vi "Incorporate New Data.vi"(8 "error in (no error)":errorcluster, 10 "New Graph Data":waveform(dbl)[](array[waveform]), 11 "Data in":T1={"UI References"={"Exit Ref"=refnum, "Save Ref"=refnum, "Open Ref"=refnum, "Export Ref"=refnum, "Acquire Ref"=refnum, "Configure Ref"=refnum, "Graph Ref"=refnum, "Clear Ref"=refnum, "Analyze Ref"=refnum, "Status Ref"=refnum, "Snapshot Ref"=refnum}, "User Specified"={"Hardware Configuration"={"VGC50"={"serial settings"={"port"="", "baud rate"=115200}, "device information"={"type"="", "model number"="", "serial number"="", "firmware version"="", "hardware version"=""}, "gauges"=[], "VGC"=refnum, "Backing SP"={"mode"=0, "thresholds"={"lower"=0.0, "upper"=0.0}, "on"=FALSE}, "Chamber SP"={"mode"=0, "thresholds"={"lower"=0.0, "upper"=0.0}, "on"=FALSE}}, "PTC10"={"serial settings"={"port"="", "baud rate"=0}, "PTC10 Info"={"Manufacturer"="", "Instrument"="", "Serial Number"="", "Firmware"=""}, "VISA resource name"=""}}, "New Data Behavior"=enum."Replace", "Vacuum Graph config"={"Log/Lin"=TRUE, "Show Backing"=FALSE, "Show Chamber"=FALSE}}} {"User Specified"."Hardware Configuration"."PTC10"."serial settings"."baud rate" items=["9600"=9600, "19200"=19200, "38400"=38400, "57600"=57600, "115200"=115200]; "User Specified"."Hardware Configuration"."VGC50"."Chamber SP"."thresholds"."upper" format="%#_5p"; "User Specified"."Hardware Configuration"."VGC50"."Chamber SP"."thresholds"."lower" format="%#_5p"; "User Specified"."Hardware Configuration"."VGC50"."Chamber SP"."mode" items=["off", "on", "channel 1", "channel 2", "channel 3"]; "User Specified"."Hardware Configuration"."VGC50"."Backing SP"."thresholds"."upper" format="%#_5p"; "User Specified"."Hardware Configuration"."VGC50"."Backing SP"."thresholds"."lower" format="%#_5p"; "User Specified"."Hardware Configuration"."VGC50"."Backing SP"."mode" items=["off", "on", "channel 1", "channel 2", "channel 3"]; "User Specified"."Hardware Configuration"."VGC50"."gauges"."status" items=["data ok", "underrange", "overrange", "sensor error", "sensor off", "no sensor", "identification error", "error BPG, HPG, BCG"]; "User Specified"."Hardware Configuration"."VGC50"."gauges"."value" format="%#_4p"; "User Specified"."Hardware Configuration"."VGC50"."serial settings"."baud rate" items=["9600"=9600, "19200"=19200, "38400"=38400, "57600"=57600, "115200"=115200]}) -> (0 "error out":errorcluster, 3 "Data out":T1={"UI References"={"Exit Ref"=refnum, "Save Ref"=refnum, "Open Ref"=refnum, "Export Ref"=refnum, "Acquire Ref"=refnum, "Configure Ref"=refnum, "Graph Ref"=refnum, "Clear Ref"=refnum, "Analyze Ref"=refnum, "Status Ref"=refnum, "Snapshot Ref"=refnum}, "User Specified"={"Hardware Configuration"={"VGC50"={"serial settings"={"port"="", "baud rate"=115200}, "device information"={"type"="", "model number"="", "serial number"="", "firmware version"="", "hardware version"=""}, "gauges"=[], "VGC"=refnum, "Backing SP"={"mode"=0, "thresholds"={"lower"=0.0, "upper"=0.0}, "on"=FALSE}, "Chamber SP"={"mode"=0, "thresholds"={"lower"=0.0, "upper"=0.0}, "on"=FALSE}}, "PTC10"={"serial settings"={"port"="", "baud rate"=0}, "PTC10 Info"={"Manufacturer"="", "Instrument"="", "Serial Number"="", "Firmware"=""}, "VISA resource name"=""}}, "New Data Behavior"=enum."Replace", "Vacuum Graph config"={"Log/Lin"=TRUE, "Show Backing"=FALSE, "Show Chamber"=FALSE}}} {"User Specified"."Hardware Configuration"."PTC10"."serial settings"."baud rate" items=["9600"=9600, "19200"=19200, "38400"=38400, "57600"=57600, "115200"=115200]; "User Specified"."Hardware Configuration"."VGC50"."Chamber SP"."thresholds"."upper" format="%#_5p"; "User Specified"."Hardware Configuration"."VGC50"."Chamber SP"."thresholds"."lower" format="%#_5p"; "User Specified"."Hardware Configuration"."VGC50"."Chamber SP"."mode" items=["off", "on", "channel 1", "channel 2", "channel 3"]; "User Specified"."Hardware Configuration"."VGC50"."Backing SP"."thresholds"."upper" format="%#_5p"; "User Specified"."Hardware Configuration"."VGC50"."Backing SP"."thresholds"."lower" format="%#_5p"; "User Specified"."Hardware Configuration"."VGC50"."Backing SP"."mode" items=["off", "on", "channel 1", "channel 2", "channel 3"]; "User Specified"."Hardware Configuration"."VGC50"."gauges"."status" items=["data ok", "underrange", "overrange", "sensor error", "sensor off", "no sensor", "identification error", "error BPG, HPG, BCG"]; "User Specified"."Hardware Configuration"."VGC50"."gauges"."value" format="%#_4p"; "User Specified"."Hardware Configuration"."VGC50"."serial settings"."baud rate" items=["9600"=9600, "19200"=19200, "38400"=38400, "57600"=57600, "115200"=115200]})   [LabVIEW 2023]
doc: "Incorporates newly acquired or loaded data into the main state data. New data can replace, be appended to, or overlayed over (as an additional channel) existing data. If the user does not have a preference saved a dialog will be presented asking which method to use."
uses:
  controls/UI References.ctl
  controls/HW Configuration.ctl
  controls/New Data Behavior.ctl
  controls/User Specified Data.ctl
  controls/Data.ctl
  controls/VGC50.ctl
  <instrlib>/PL Inficon VGC/PL Inficon VGC.lvclass
  controls/SRS PTC10.ctl
  controls/Vac Graph Config.ctl
panel:
  # "(Scroll up to see large state data in/out clusters)"
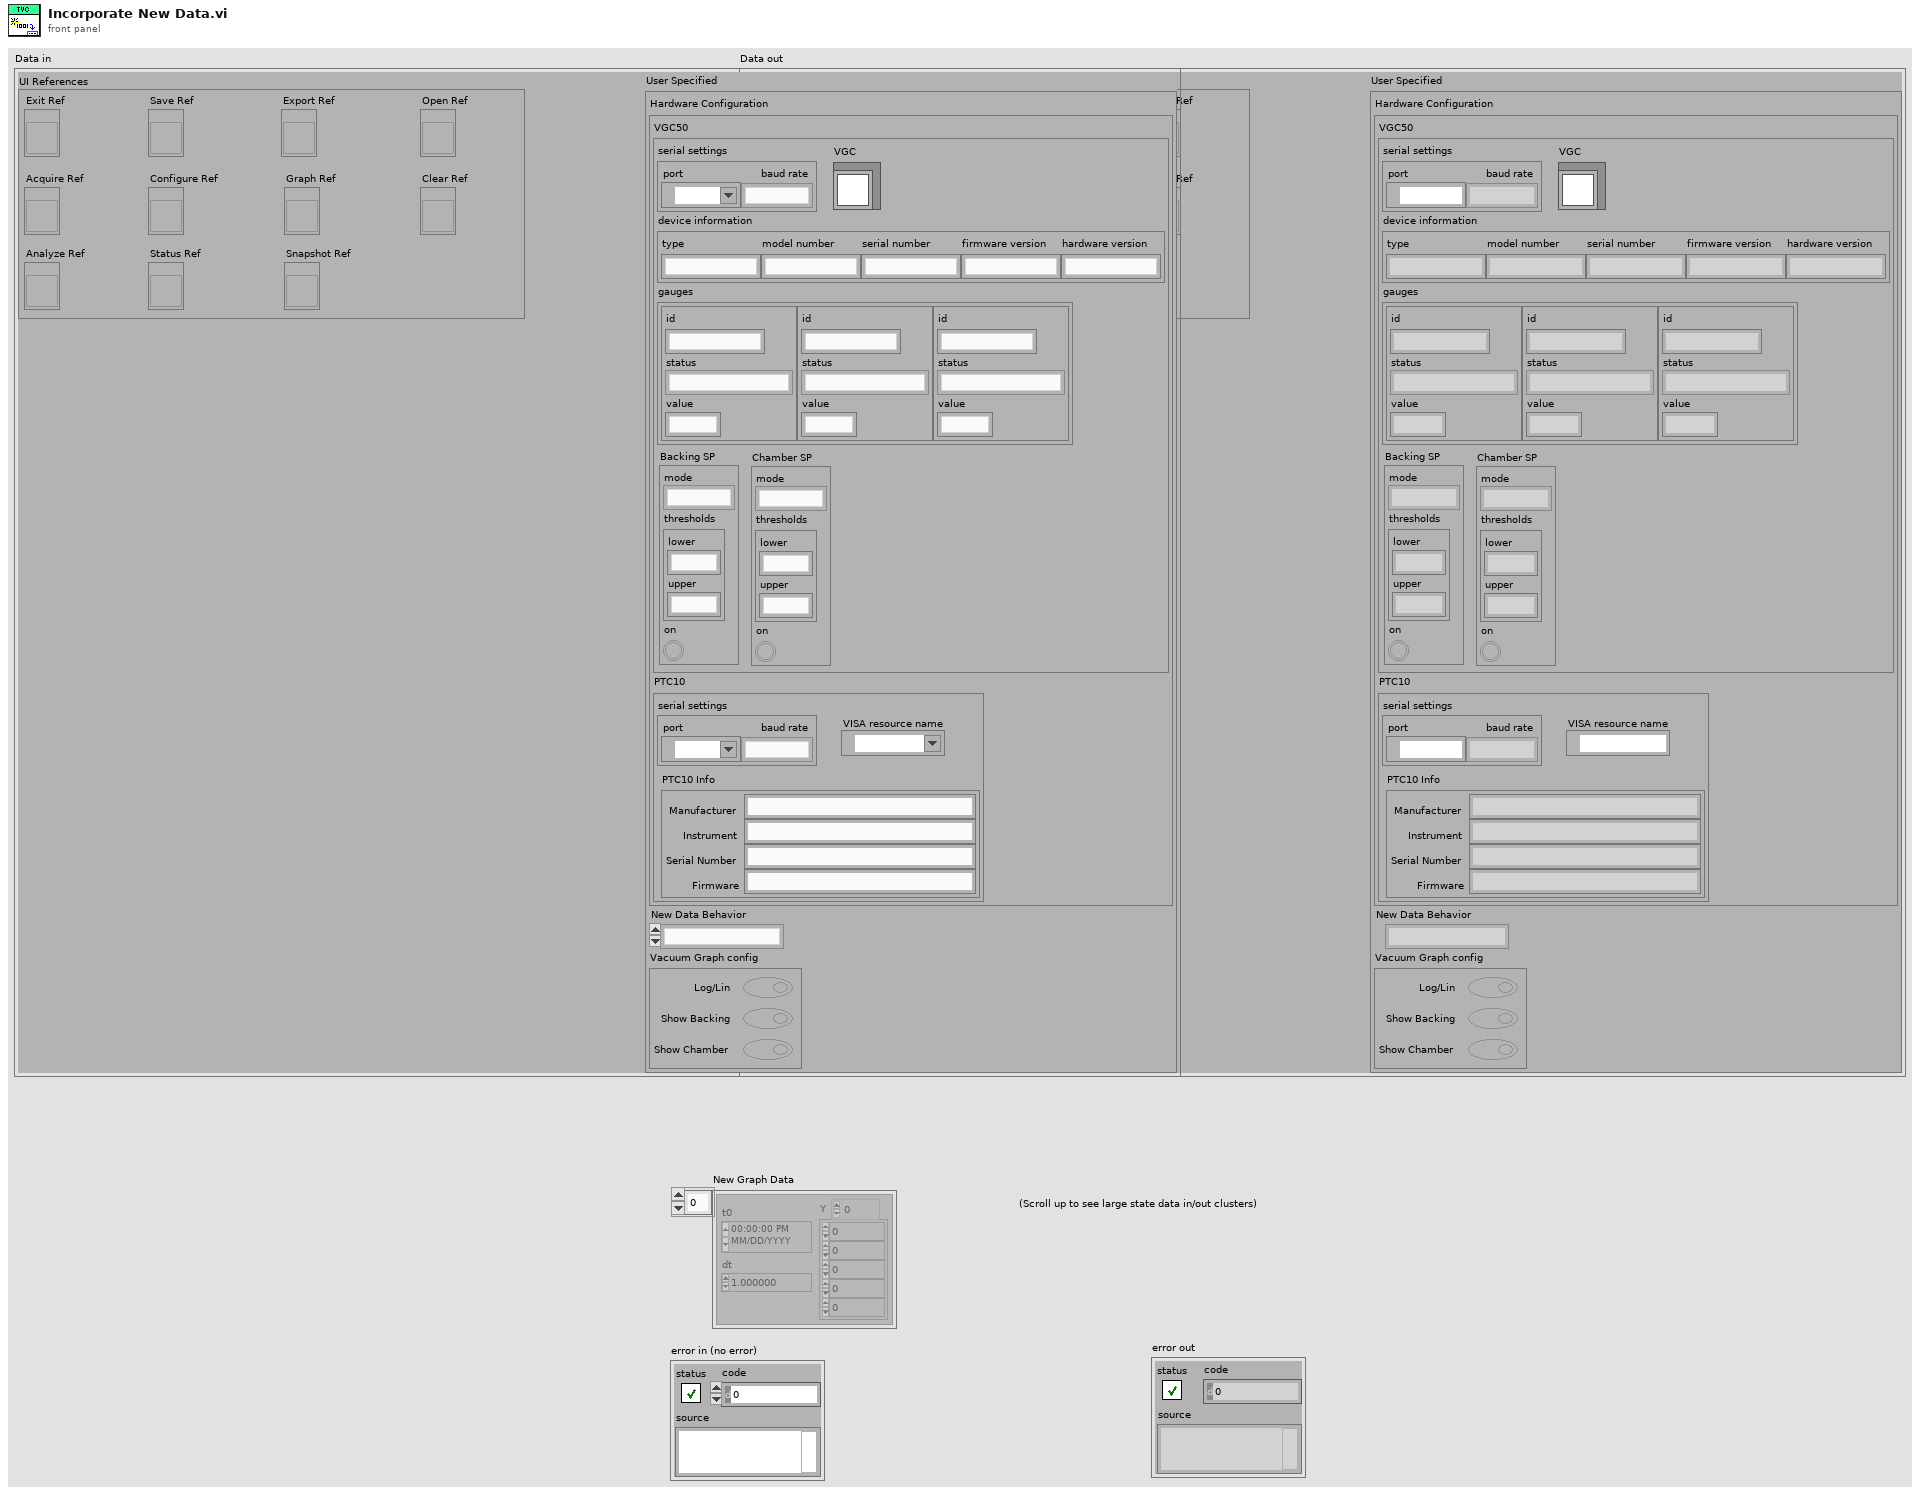
[diagram p1: front panel]
types:
  T1 = typedef "Data.ctl" = cluster{"UI References":T2, "User Specified":T3}
  T2 = typedef "UI References.ctl" = cluster{"Exit Ref":refnum<vi>, "Save Ref":refnum<vi>, "Open Ref":refnum<vi>, "Export Ref":refnum<vi>, "Acquire Ref":refnum<vi>, "Configure Ref":refnum<vi>, "Graph Ref":refnum<vi>, "Clear Ref":refnum<vi>, "Analyze Ref":refnum<vi>, "Status Ref":refnum<vi>, "Snapshot Ref":refnum<vi>}
  T3 = typedef "User Specified Data.ctl" = cluster{"Hardware Configuration":T4, "New Data Behavior":T7, "Vacuum Graph config":T8}
  T4 = typedef "HW Configuration.ctl" = cluster{"VGC50":T5, "PTC10":T6}
  T5 = typedef "VGC50.ctl" = cluster{"serial settings":cluster{"port":refnum<visa-resource-name>, "baud rate":u32}, "device information":cluster{"type":string, "model number":string, "serial number":string, "firmware version":string, "hardware version":string}, "gauges":cluster{"id":string, "status":u16, "value":dbl}[], "VGC":refnum<class "PL Inficon VGC.lvclass">, "Backing SP":cluster{"mode":u16, "thresholds":cluster{"lower":dbl, "upper":dbl}, "on":bool}, "Chamber SP":cluster{"mode":u16, "thresholds":cluster{"lower":dbl, "upper":dbl}, "on":bool}}
  T6 = typedef "SRS PTC10.ctl" = cluster{"serial settings":cluster{"port":refnum<visa-resource-name>, "baud rate":u32}, "PTC10 Info":cluster{"Manufacturer":string, "Instrument":string, "Serial Number":string, "Firmware":string}, "VISA resource name":refnum<visa-resource-name>}
  T7 = typedef "New Data Behavior.ctl" = enum16{"Replace", "Overlay", "Append"}
  T8 = typedef "Vac Graph Config.ctl" = cluster{"Log/Lin":bool, "Show Backing":bool, "Show Chamber":bool}
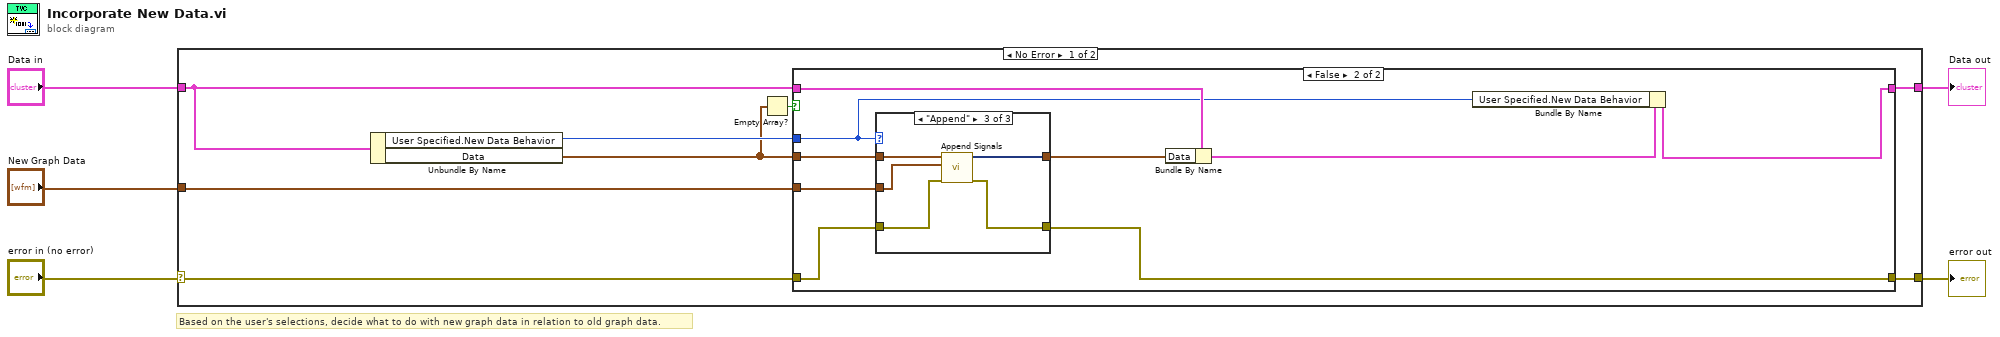
[diagram p0: block diagram]
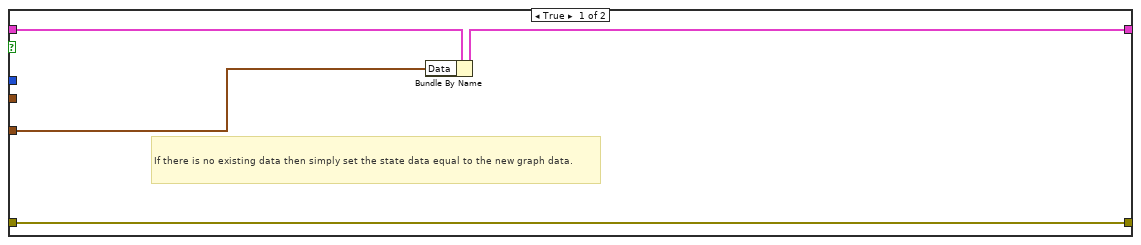
[diagram p2: hidden frame]
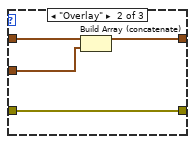
[diagram p4: hidden frame]
diagram:
  # "Based on the user's selections, decide what to do with new graph data in relation to old graph data."
  n1 = case shown="No Error" "error in (no error)" {
    selector: "error in (no error)" -> [w9 w39]
    tunnel: "Data in" -> [w13 w38]
    tunnel: "New Graph Data" -> [w11 _]
    tunnel: [w10 w38] -> w3
    tunnel: [w8 w39] -> w1
    frame No Error {
      n2 = Unbundle By Name(w13) -> ("User Specified.New Data Behavior"=w12:T7, "Data"=w7:waveform(dbl)[])
      n3 = Empty Array?(array=w7) -> (empty?=w6:bool)
      n4 = case shown="False" w6 {
        tunnel: w13 -> [w17 w26]
        tunnel: w12 -> [_ w18]
        tunnel: w11 -> [w16 w25]
        tunnel: w7 -> [_ w23]
        tunnel: [w15 w21] -> w10
        tunnel: w9 -> [w14 w20]
        tunnel: [w14 w19] -> w8
        frame True {
          # "If there is no existing data then simply set the state data equal to the new graph data."
          n5 = Bundle By Name(cluster=w17, "Data"=w16) -> (w15:T1)
        }
        frame False {
          n6 = case shown="\"Append\"" w18 {
            tunnel: w25 -> [w28 w31 w36]
            tunnel: [w28 w30 w35] -> w24
            tunnel: w23 -> [_ w32 w37]
            tunnel: w20 -> [w27 w29 w34]
            tunnel: [w27 w29 w33] -> w19
            frame "Replace" {
            }
            frame "Overlay" {
              n7 = Build Array (concatenate)(w32, w31) -> (w30:waveform(dbl)[])
            }
            frame "Append" {
              n8 = call "Append Signals"("error in (no error)"=w34, "Input Signal B"=w36, "Input Signal A"=w37) -> ("error out"=w33:errorcluster, "Appended Signals"=w35:dynamicdata)  [unwired: 7 in]
            }
          }
          n9 = Bundle By Name(cluster=w26, "Data"=w24) -> (w22:T1)
          n10 = Bundle By Name(cluster=w22, "User Specified.New Data Behavior"=w18) -> (w21:T1)
        }
      }
    }
    frame Error {
    }
  }
  "Data out" <- w3
  "error out" <- w1
